vi "Get_User_Anwers.vi"(0 "Application_Directory":path, 11 "Error_In":errorcluster) -> (4 "User_Answer":string[](array[string]), 15 "Error_Out":errorcluster)   [LabVIEW 2023]
doc: "This VI gets the user asnwers form ini."
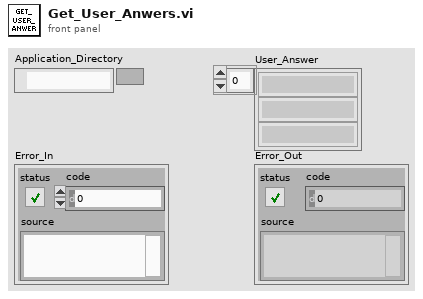
[diagram p1: front panel]
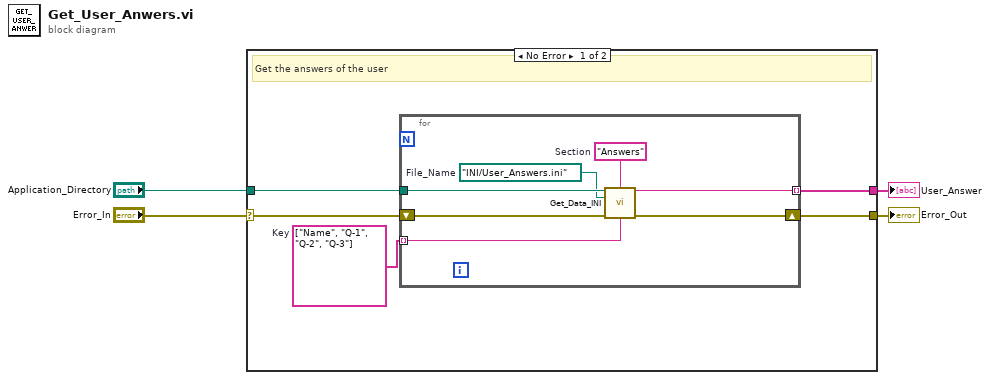
[diagram p0: block diagram]
diagram:
  n1 = case shown="No Error" "Error_In" {
    selector: "Error_In" -> [w6 w17]
    tunnel: [w9 w17] -> w3
    tunnel: "Application_Directory" -> [w8 _]
    tunnel: [w5 _] -> w2
    frame No Error {
      w7 = string[] ["Name", "Q-1", "Q-2", "Q-3"]  # Key
      # "Get the answers of the user"
      n2 = for {
        tunnel: w8 -> [w14]
        shift-right: [w15] -> w9
        shift-left: w6 -> [w16]
        tunnel: w7 -> [w11] mode=indexing
        tunnel: [w10] -> w5 mode=indexing
        w12 = "Answers"  # Section
        w13 = path "INI/User_Answers.ini"  # File_Name
        n3 = call "Get_Data_INI.vi"("Application_Directory"=w14, "Section"=w12, "File_Name"=w13, "Error_In"=w16, "Key"=w11) -> ("Data"=w10:string, "Error_Out"=w15:errorcluster)  [unwired: 9 in]
      }
    }
    frame Error {
    }
  }
  "Error_Out" <- w3
  "User_Answer" <- w2
